vi "ReloadPositionsTest.vi"() -> ()   [LabVIEW 2013]
panel:
  out "Array":string[](array[string])
  in  "Load Positions":dbl[](array[numeric])
  out "IP 2":string caption="Custom Command: Response"
  out "Positions 2":i32[](array[numeric])
  out "Positions":i32[](array[numeric])
  out "IP":string caption="Custom Command: Response"
  out "error out":errorcluster
  in  "PicoMotor IP":string="192.168.14.151"
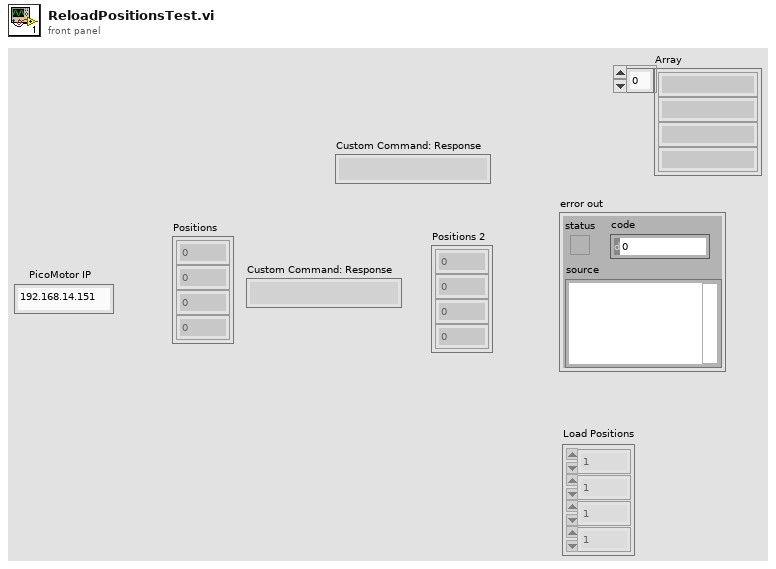
[diagram p1: front panel]
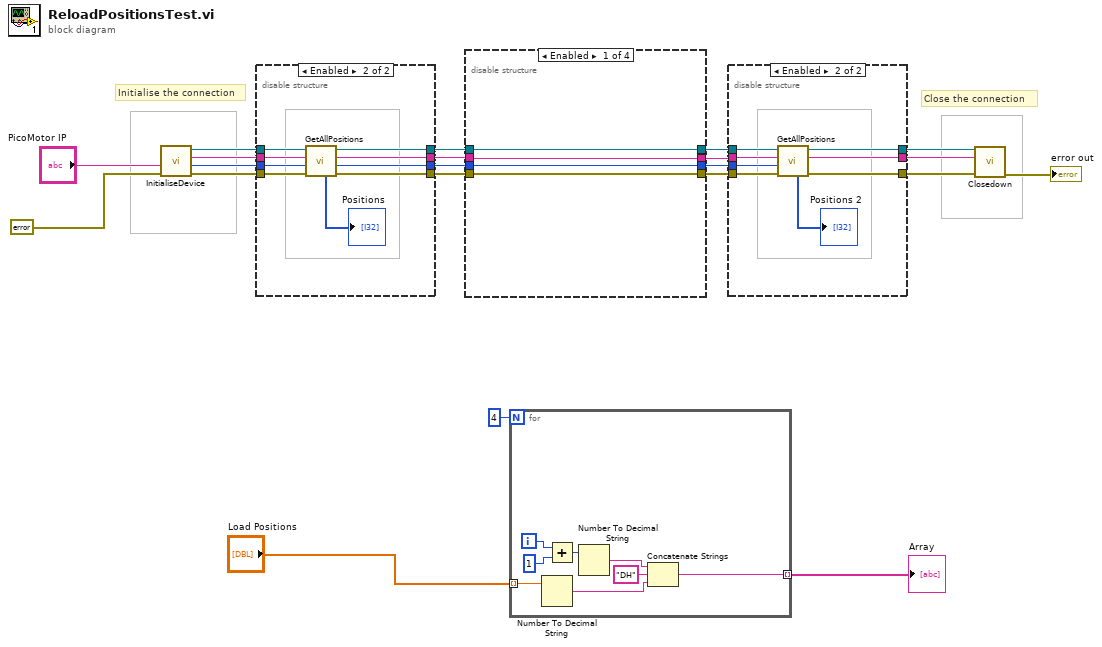
[diagram p0: block diagram]
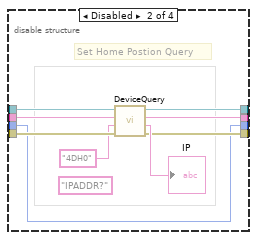
[diagram p3: hidden frame]
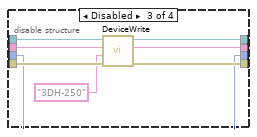
[diagram p4: hidden frame]
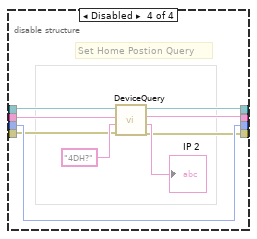
[diagram p5: hidden frame]
diagram:
  # "Close the connection"
  # "Initialise the connection"
  n1 = call "InitialiseDevice.vi"("error In"=errorcluster {"status"=FALSE, "code"=0, "source"=""}, "PicoMotor IP In"="PicoMotor IP") -> ("error out"=w16:errorcluster, "Device Address Out"=w17:i32, "DeviceKey Out"=w18:string, "CmdLib Out"=w19:refnum<k24>)  [unwired: 6 in]
  n2 = disable-structure shown="Enabled" {
    disable-tunnel: w19 -> [w24 w29]
    disable-tunnel: w18 -> [w23 w30]
    disable-tunnel: w17 -> [_ w31]
    disable-tunnel: w16 -> [w22 w32]
    disable-tunnel: [w22 w26] -> w14
    disable-tunnel: [w24 w28] -> w13
    disable-tunnel: [w23 w27] -> w12
    disable-tunnel: [_ w25] -> w4
    frame Disabled {
    }
    frame Enabled {
      n3 = call "GetAllPositions.vi"("error In"=w32, "Device Address In"=w31, "DeviceKey In"=w30, "CmdLib In"=w29) -> ("error out"=w26:errorcluster, "Device Address Out"=w25:i32, "DeviceKey Out"=w27:string, "CmdLib Out"=w28:refnum<k24>, "Positions"=→"Positions":i32[])  [unwired: 3 in]
    }
  }
  n4 = disable-structure shown="Enabled" {
    disable-tunnel: [w37 w41 w51 w60] -> w11
    disable-tunnel: [w36 w42 w50 w57] -> w10
    disable-tunnel: [w35 w43 w52 w56] -> w9
    disable-tunnel: w14 -> [w35 w44 w53 w55]
    disable-tunnel: w13 -> [w37 w40 w54 w59]
    disable-tunnel: w12 -> [w36 w45 w49 w58]
    disable-tunnel: [w34 w39 w48 w61] -> w5
    disable-tunnel: w4 -> [w34 w39 w48 w61]
    frame Enabled {
    }
    frame Disabled {
      (unwired) "IPADDR?"
      # "Set Home Postion Query"
      n5 = call "DeviceQuery.vi"("error in (no error)"=w44, "Command"="4DH0", "DeviceKey In"=w45, "CmdLib In"=w40) -> ("error out"=w43:errorcluster, "Response"=→"IP":string, "DeviceKey Out"=w42:string, "CmdLib Out"=w41:refnum<k24>)
    }
    frame Disabled {
      n6 = call "DeviceWrite.vi"("error in (no error)"=w53, "Command"="3DH-250", "DeviceKey In"=w49, "CmdLib In"=w54) -> ("error out"=w52:errorcluster, "DeviceKey Out"=w50:string, "CmdLib Out"=w51:refnum<k24>)  [unwired: 1 in]
    }
    frame Disabled {
      # "Set Home Postion Query"
      n7 = call "DeviceQuery.vi"("error in (no error)"=w55, "Command"="4DH?", "DeviceKey In"=w58, "CmdLib In"=w59) -> ("error out"=w56:errorcluster, "Response"=→"IP 2":string, "DeviceKey Out"=w57:string, "CmdLib Out"=w60:refnum<k24>)
    }
  }
  n8 = for {
    N: 4 -> [_]
    tunnel: [w69] -> w2 mode=indexing
    tunnel: "Load Positions" -> [w64] mode=indexing
    i -> [w67]
    n9 = Number To Decimal String(number=w64) -> (decimal integer string=w65:string)  [unwired: 1 in]
    n10 = Add(x=w67, y=1) -> (x+y=w68:i32)
    n11 = Number To Decimal String(number=w68) -> (decimal integer string=w71:string)  [unwired: 1 in]
    n12 = Concatenate Strings(w71, "DH" ("string"), w65) -> (w69:string)
  }
  "Array" <- w2
  n13 = disable-structure shown="Enabled" {
    disable-tunnel: w11 -> [w74 w78]
    disable-tunnel: w10 -> [w73 w79]
    disable-tunnel: w5 -> [_ w80]
    disable-tunnel: w9 -> [w72 w81]
    disable-tunnel: [w72 w75] -> w8
    disable-tunnel: [w74 w77] -> w6
    disable-tunnel: [w73 w76] -> w7
    frame Disabled {
    }
    frame Enabled {
      n14 = call "GetAllPositions.vi"("error In"=w81, "Device Address In"=w80, "DeviceKey In"=w79, "CmdLib In"=w78) -> ("error out"=w75:errorcluster, "DeviceKey Out"=w76:string, "CmdLib Out"=w77:refnum<k24>, "Positions"=→"Positions 2":i32[])  [unwired: 3 in, 1 out]
    }
  }
  n15 = call "Closedown.vi"("error In"=w8, "DeviceKey In"=w7, "CmdLib In"=w6) -> ("error out"=→"error out":errorcluster)  [unwired: 8 in]
